vi "Parse Relative Flow.vi"() -> ()   [LabVIEW 2010]
panel:
  in  "Flow Command":string="<3.5>+175.3"
  in  "error in":errorcluster
  out "error out":errorcluster
  out "Flow Value to Add to Reference":dbl
  out "Step Reference":i32
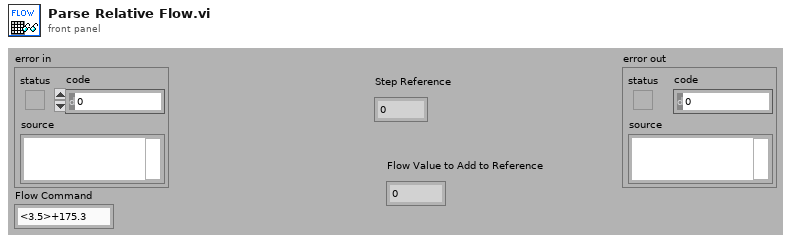
[diagram p1: front panel]
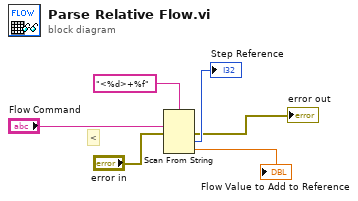
[diagram p0: block diagram]
diagram:
  # "<"
  n1 = Scan From String(format string="<%d>+%f", input string="Flow Command", error in="error in") -> (error out=→"error out":errorcluster, output 1=→"Step Reference":i32, output 2=→"Flow Value to Add to Reference":dbl)  [unwired: 3 in, 2 out]
